vi "Publisher-TCSS.vi"(9 "buttonSend":bool, 10 "OSS_Supervisory":T1) -> ()   [LabVIEW 2019]
uses:
  OSS_Supervisory.ctl
  <vilib>/Distrio/LabbitMQ/Connection/Connection.lvclass
  <vilib>/Distrio/LabbitMQ/Connection/connection_parameters_cluster.ctl
  <vilib>/Distrio/LabbitMQ/Channel/exchange_type_enum.ctl
  <vilib>/Distrio/LabbitMQ/Exchange/Exchange.lvclass
  <vilib>/Distrio/LabbitMQ/Channel/Channel.lvclass
panel:
  in  "buttonStop":bool
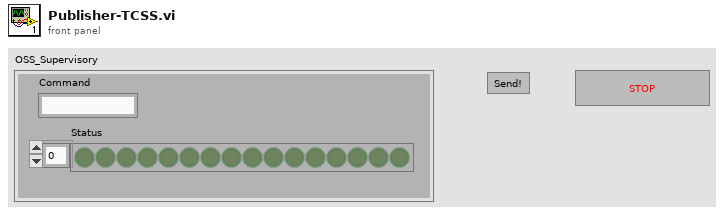
[diagram p1: front panel]
types:
  T1 = typedef "OSS_Supervisory.ctl" = cluster{"Command":string, "Status":bool[]}
  T2 = typedef "Connection.lvclass/connection_parameters_cluster.ctl" = cluster{"host name":string, "port":i32, "user name":string, "password":string, "virtual host":string}
  T3 = typedef "Channel.lvclass/exchange_type_enum.ctl" = enum16{"direct", "topic", "fanout", "headers"}
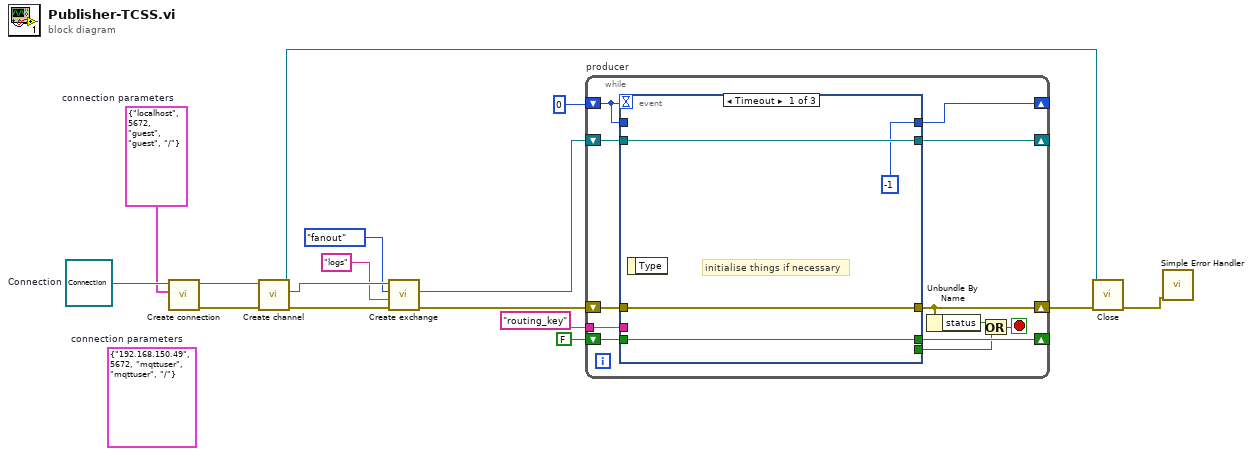
[diagram p0: block diagram]
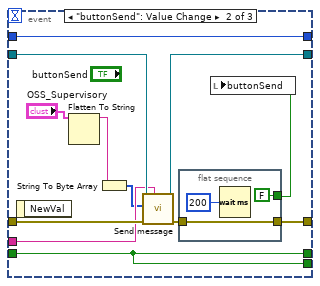
[diagram p2: hidden frame]
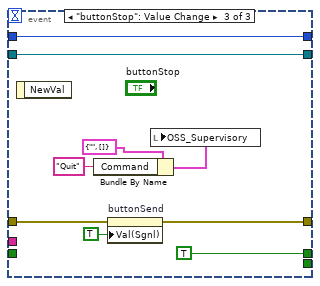
[diagram p3: hidden frame]
diagram:
  (unwired) T2 {"host name"="192.168.150.49", "port"=5672, "user name"="mqttuser", "password"="mqttuser", "virtual host"="/"}  # connection parameters
  w4 = T2 {"host name"="localhost", "port"=5672, "user name"="guest", "password"="guest", "virtual host"="/"}  # connection parameters
  w14 = refnum<class "Connection.lvclass"> refnum  # Connection
  n1 = call <vilib>:"Create connection.vi"("connection parameters"=w4, "Connection in"=w14) -> ("error out"=w10:errorcluster, "Connection out"=w9:refnum<class "Connection.lvclass">)  [unwired: 8 in]
  n2 = call <vilib>:"Create channel.vi"("error in (no error)"=w10, "Connection in"=w9) -> ("error out"=w7:errorcluster, "channel"=w8:refnum<class "Channel.lvclass">, "Connection out"=w12:refnum<class "Connection.lvclass">)  [unwired: 7 in]
  n3 = call <vilib>:"Create exchange.vi"("error in (no error)"=w7, "exchange name"="logs", "exchange type"=exchange_type_enum."fanout" ("binding"), "Channel in"=w8) -> ("error out"=w6:errorcluster, "Exchange.lvclass"=w5:refnum<class "Exchange.lvclass">)  [unwired: 5 in, 1 out]
  n4 = while "producer" {
    shift-right: [w26] -> w11
    shift-left: w6 -> [w27]
    shift-right: [w25] -> _
    shift-left: w5 -> [w28]
    shift-right: [w18] -> _
    shift-left: FALSE -> [w22]
    tunnel: "routing_key" -> [w21]
    shift-right: [w19] -> _
    shift-left: 0 -> [w20]
    stop <- w23 stop-if-true
    n5 = event shown="[0] Timeout" {
      selector: _ -> [_ _ _]
      dyn-events: _ -> [_ _ _]
      timeout: w20 -> [_ _ _]
      tunnel: w28 -> [w32 w40 w56]
      tunnel: w27 -> [w31 w42 w54]
      tunnel: [w31 w37 w53] -> w26
      tunnel: [w32 w41 w56] -> w25
      tunnel: w22 -> [w30 w43 _]
      tunnel: [w30 w43 TRUE] -> w18
      tunnel: w21 -> [_ w39 _]
      tunnel: w20 -> [_ w44 w51]
      tunnel: [-1 w44 w51] -> w19
      tunnel: [_ w43 _] -> w17
      event Timeout {
        # "initialise things if necessary"
        n6 = event-data() -> ()  [unwired: 1 in, 1 out]
      }
      event "buttonSend": Value Change {
        n7 = event-data() -> ()  [unwired: 1 in, 1 out]
        n8 = Flatten To String(anything="OSS_Supervisory") -> (data string=w34:string)  [unwired: 3 in, 2 out]
        n9 = String To Byte Array(string=w34) -> (unsigned byte array=w35:u8[])
        n10 = call <vilib>:"Send message.vi"("routing key"=w39, "error in (no error)"=w42, "body"=w35, "Exchange in"=w40) -> ("error out"=w38:errorcluster, "Exchange out"=w41:refnum<class "Exchange.lvclass">)  [unwired: 6 in]
        n11 = flat-sequence {
          tunnel: w38 -> [w46]
          tunnel: [w46] -> w37
          tunnel: [FALSE ("buttonSend")] -> w36
          frame #0 {
            n12 = Wait (ms)(milliseconds to wait=u32 200) -> ()  [unwired: 1 out]
          }
        }
        n13 = local write "buttonSend"(w36) -> ()
      }
      event "buttonStop": Value Change {
        n14 = event-data() -> ()  [unwired: 1 in, 1 out]
        n15 = Bundle By Name(cluster=cluster{"Command":string, "Status":bool[]} {"Command"="", "Status"=[]} ("OSS_Supervisory"), "Command"="Quit") -> (w50:cluster{"Command":string, "Status":bool[]})
        n16 = property on="buttonSend" class="Bool (strict)"(error in=w54, "Val(Sgnl)"=TRUE ("Value (Signaling)")) -> (error out=w53:errorcluster)  [unwired: 1 in, 1 out]
        n17 = local write "OSS_Supervisory"(w50) -> ()
      }
    }
    n18 = Unbundle By Name(w26) -> ("status"=w24:bool)
    n19 = Or(x=w24, y=w17) -> (x .or. y?=w23:bool)
  }
  n20 = call <vilib>:"Close.vi"("error in (no error)"=w11, "Connection in"=w12) -> ("error out"=w1:errorcluster)  [unwired: 8 in, 1 out]
  n21 = call <vilib>:"Simple Error Handler.vi"("error in (no error)"=w1) -> ()  [unwired: 4 in, 5 out]
